vi "Wrapper.vi"   [LabVIEW 2019]
uses:
  Protocols.lvlib
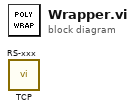
[diagram p0: block diagram]
diagram:
  n1 = call "TCP.vi"() -> ()  [unwired: 12 in]
  n2 = call "RS-xxx.vi"() -> ()  [unwired: 12 in]
